vi "SortData.vi"(10 "SortBy":enum16{"Name", "Number", "Producer"}(ring), 11 "ProductsToSort":T1[](array[typedef])) -> (3 "ProductsSorted":T1[](array[typedef]))   [LabVIEW 2018]
uses:
  ProductsCluster.ctl
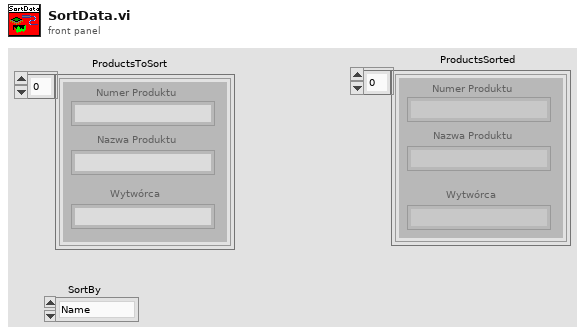
[diagram p1: front panel]
types:
  T1 = typedef "ProductsCluster.ctl" = cluster{"Numer Produktu":string, "Nazwa Produktu":string, "Wytwórca":string}
  T2 = cluster{"Nazwa Produktu":string, "ProgramData":T1}
  T3 = cluster{"Numer Produktu":string, "ProgramData":T1}
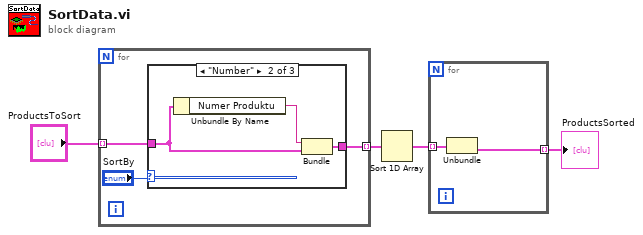
[diagram p0: block diagram]
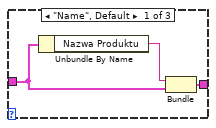
[diagram p2: hidden frame]
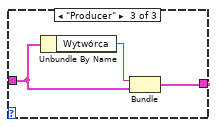
[diagram p3: hidden frame]
diagram:
  n1 = for {
    tunnel: "ProductsToSort" -> [w7] mode=indexing
    tunnel: [w6] -> w3 mode=indexing
    n2 = case shown="\"Number\"" "SortBy" {
      tunnel: w7 -> [w9 w12 w14]
      tunnel: [w8 w13 w15] -> w6
      frame "Name", Default {
        n3 = Unbundle By Name(w9) -> ("Nazwa Produktu"=w10:string)
        n4 = Bundle("Nazwa Produktu"=w10, "ProgramData"=w9) -> (w8:T2)  [unwired: 1 in]
      }
      frame "Number" {
        n5 = Unbundle By Name(w12) -> ("Numer Produktu"=w11:string)
        n6 = Bundle("Numer Produktu"=w11, "ProgramData"=w12) -> (w13:T3)  [unwired: 1 in]
      }
      frame "Producer" {
        n7 = Unbundle By Name(w14) -> ("Wytwórca"=w16:string)
        n8 = Bundle("Wytwórca"=w16, "ProgramData"=w14) -> (w15:cluster{"Wytwórca":string, "ProgramData":T1})  [unwired: 1 in]
      }
    }
  }
  n9 = Sort 1D Array(array=w3) -> (sorted array=w4:cluster{"Wytwórca":string, "ProgramData":T1}[])
  n10 = for {
    tunnel: w4 -> [w18] mode=indexing
    tunnel: [w17] -> w1 mode=indexing
    n11 = Unbundle(w18) -> ("ProgramData"=w17:T1)  [unwired: 1 out]
  }
  "ProductsSorted" <- w1
